vi "parse serial data.vi"(8 "serial data":dbl[][](array[numeric])) -> (0 "coil data":T1[](array[typedef]), 1 "mag data":T2[](array[typedef]), 2 "accel data":T2[](array[typedef]), 3 "voltage data":T1[](array[typedef]))   [LabVIEW 2017]
uses:
  typedefs/reading3.ctl
  typedefs/reading1.ctl
  typedefs/readingType.ctl
  9d131113-3482-4a79-8b18-faa5a8e8f46f.vi
  <vilib>/Array/Sort 2D Array - Pop Stack.vi
  <vilib>/Array/Sort 2D Array - Push Stack.vi
  9d131113-3482-4a79-8b18-faa5a8e8f46f.vi/677e4750-3293-40eb-b03c-131809e5ca16.vi
panel:
  out "max(x,y)":dbl
  out "min value":dbl
  out "max value":dbl
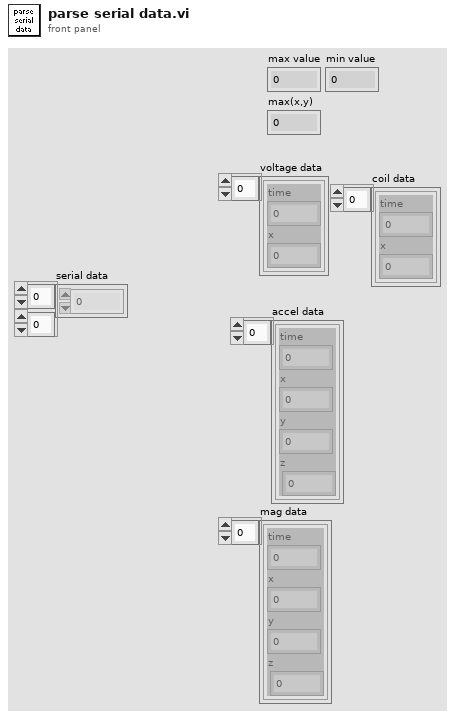
[diagram p1: front panel]
types:
  T1 = typedef "reading1.ctl" = cluster{"time":dbl, "x":dbl}
  T2 = typedef "reading3.ctl" = cluster{"time":dbl, "x":dbl, "y":dbl, "z":dbl}
  T3 = typedef "readingType.ctl" = enum16{"none", "analogV", "magx", "magy", "magz", "accx", "accy", "accz", "coil"}
  T4 = enum16{"none", "analogV", "magx", "magy", "magz", "accx", "accy", "accz"}
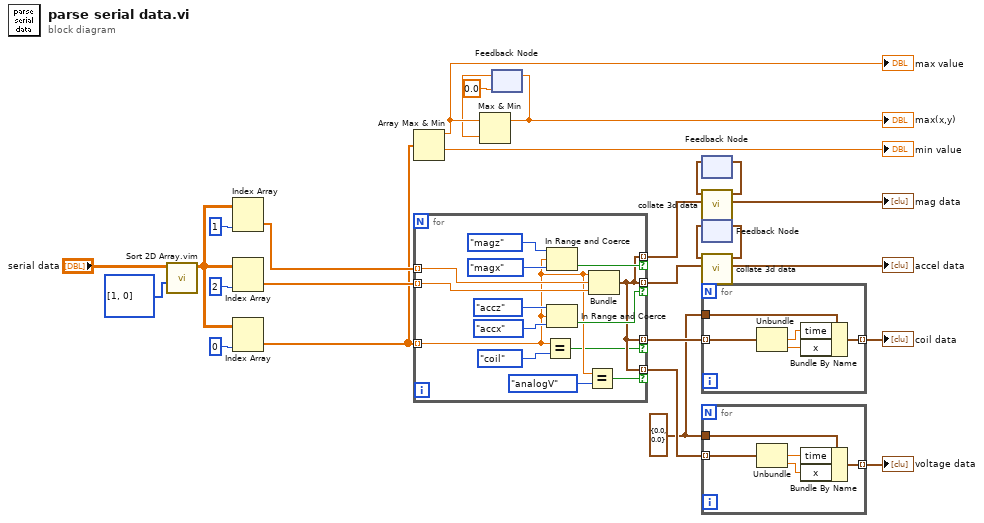
[diagram p0: block diagram]
diagram:
  w12 = T1 {"time"=0.0, "x"=0.0} ("reading1")
  n1 = call "Sort 2D Array.vim"("index"=i32[] [1, 0], "2D array"="serial data") -> ("sorted 2D array"=w21:dbl[][])  [unwired: 8 in, 1 out]
  n2 = Index Array(array=w21, index (col)=1 ("disabled index (col)")) -> (element=w24:dbl[])  [unwired: 1 in]
  n3 = Index Array(array=w21, index (col)=2 ("disabled index (col)")) -> (element=w23:dbl[])  [unwired: 1 in]
  n4 = Index Array(array=w21, index (col)=0 ("disabled index (col)")) -> (element=w10:dbl[])  [unwired: 1 in]
  n5 = Array Max & Min(array=w10) -> (max value=w8:dbl, min value=→"min value":dbl)  [unwired: 2 out]
  "max value" <- w8
  n6 = for {
    tunnel: w10 -> [w31] mode=indexing
    tunnel: w24 -> [w41] mode=indexing
    tunnel: w23 -> [w40] mode=indexing
    tunnel: [w32] -> w15 mode=indexing if=w33
    tunnel: [w32] -> w19 mode=indexing if=w35
    tunnel: [w32] -> w18 mode=indexing if=w34
    tunnel: [w32] -> w13 mode=indexing if=w28
    n7 = Equal?(x=w31, y=readingType."coil" ("reading type")) -> (x = y?=w28:bool)
    n8 = In Range and Coerce(upper limit=T4."magz" ("reading type"), x=w31, lower limit=T4."magx" ("reading type")) -> (In Range?=w35:bool)  [unwired: 1 out]
    n9 = In Range and Coerce(upper limit=T4."accz" ("reading type"), x=w31, lower limit=T4."accx" ("reading type")) -> (In Range?=w34:bool)  [unwired: 1 out]
    n10 = Equal?(x=w31, y=readingType."analogV" ("reading type")) -> (x = y?=w33:bool)
    n11 = Bundle(w31, w41, w40) -> (w32:cluster{dbl, dbl, dbl})  [unwired: 1 in]
  }
  n12 = feedback #1(0.0) -> (w6:dbl)
  n13 = Max & Min(x=w8, y=w6) -> (max(x,y)=w7:dbl)  [unwired: 1 out]
  "max(x,y)" <- w7
  n14 = feedback-in #1(w7) -> ()
  n15 = feedback #2() -> (w3:cluster{"type":dbl, "time":dbl, "data":dbl}[])  [unwired: 1 in]
  n16 = call "collate 3d data.vi"("sorted input data"=w19, "leftover"=w3) -> ("3d vs t data"=→"mag data":T2[], "leftover to feedback"=w4:cluster{"type":dbl, "time":dbl, "data":dbl}[])  [unwired: 8 in]
  n17 = feedback-in #2(w4) -> ()
  n18 = feedback #3() -> (w1:cluster{"type":dbl, "time":dbl, "data":dbl}[])  [unwired: 1 in]
  n19 = call "collate 3d data.vi"("sorted input data"=w18, "leftover"=w1) -> ("3d vs t data"=→"accel data":T2[], "leftover to feedback"=w2:cluster{"type":dbl, "time":dbl, "data":dbl}[])  [unwired: 8 in]
  n20 = feedback-in #3(w2) -> ()
  n21 = for {
    tunnel: w13 -> [w46] mode=indexing
    tunnel: w12 -> [w45]
    tunnel: [w42] -> w11 mode=indexing
    n22 = Unbundle(w46) -> (w44:dbl, w43:dbl)  [unwired: 1 out]
    n23 = Bundle By Name(cluster=w45, "time"=w44, "x"=w43) -> (w42:T1)
  }
  "coil data" <- w11
  n24 = for {
    tunnel: w15 -> [w51] mode=indexing
    tunnel: w12 -> [w50]
    tunnel: [w47] -> w14 mode=indexing
    n25 = Unbundle(w51) -> (w49:dbl, w48:dbl)  [unwired: 1 out]
    n26 = Bundle By Name(cluster=w50, "time"=w49, "x"=w48) -> (w47:T1)
  }
  "voltage data" <- w14
